vi "性能模式.vi"(7 "colomn":string, 11 "数据标识输入":string) -> (3 "数据标识输出":string)   [LabVIEW 2016]
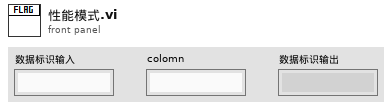
[diagram p1: front panel]
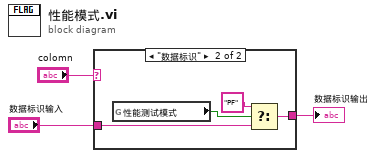
[diagram p0: block diagram]
diagram:
  n1 = case shown="\"数据标识\"" "colomn" {
    tunnel: [w4 w8] -> w3
    tunnel: "数据标识输入" -> [w4 w7]
    frame Default {
    }
    frame "数据标识" {
      n2 = global read "外部调用接口全局变量.vi" "性能测试模式"() -> (w5:bool)
      n3 = Select(t="PF", s=w5, f=w7) -> (s? t:f=w8:string)
    }
  }
  "数据标识输出" <- w3
